vi "Untitled 1 (SubVI).vi"(5 "Sensor Data":string[][](array[string]), 6 "LDO Control Input":T3, 7 "Data Cluster":T5, 8 "error in (no error)":errorcluster, 9 "Ultramat 23":string[][](array[string]), 10 "Gross Heating Value, Vol (Real, Dry)":dbl, 11 "Header Array":string[](array[string])) -> (0 "error out":errorcluster, 2 "Gas Rate (BTU/hr)":dbl, 3 "Array":string[][](array[string]))   [LabVIEW 2020]
uses:
  Modbus LDO Control.ctl
  Drivers/Alicat LabVIEW Drivers 2v1/Sub-VIs/Data Cluster.ctl
  Modbus PLC Data All.ctl
  Modbus FVIR Control.ctl
  WritingDataFile/Data to Save.ctl
panel:
  in  "PLC Data Out":T1
  # "Totalizer Timer"
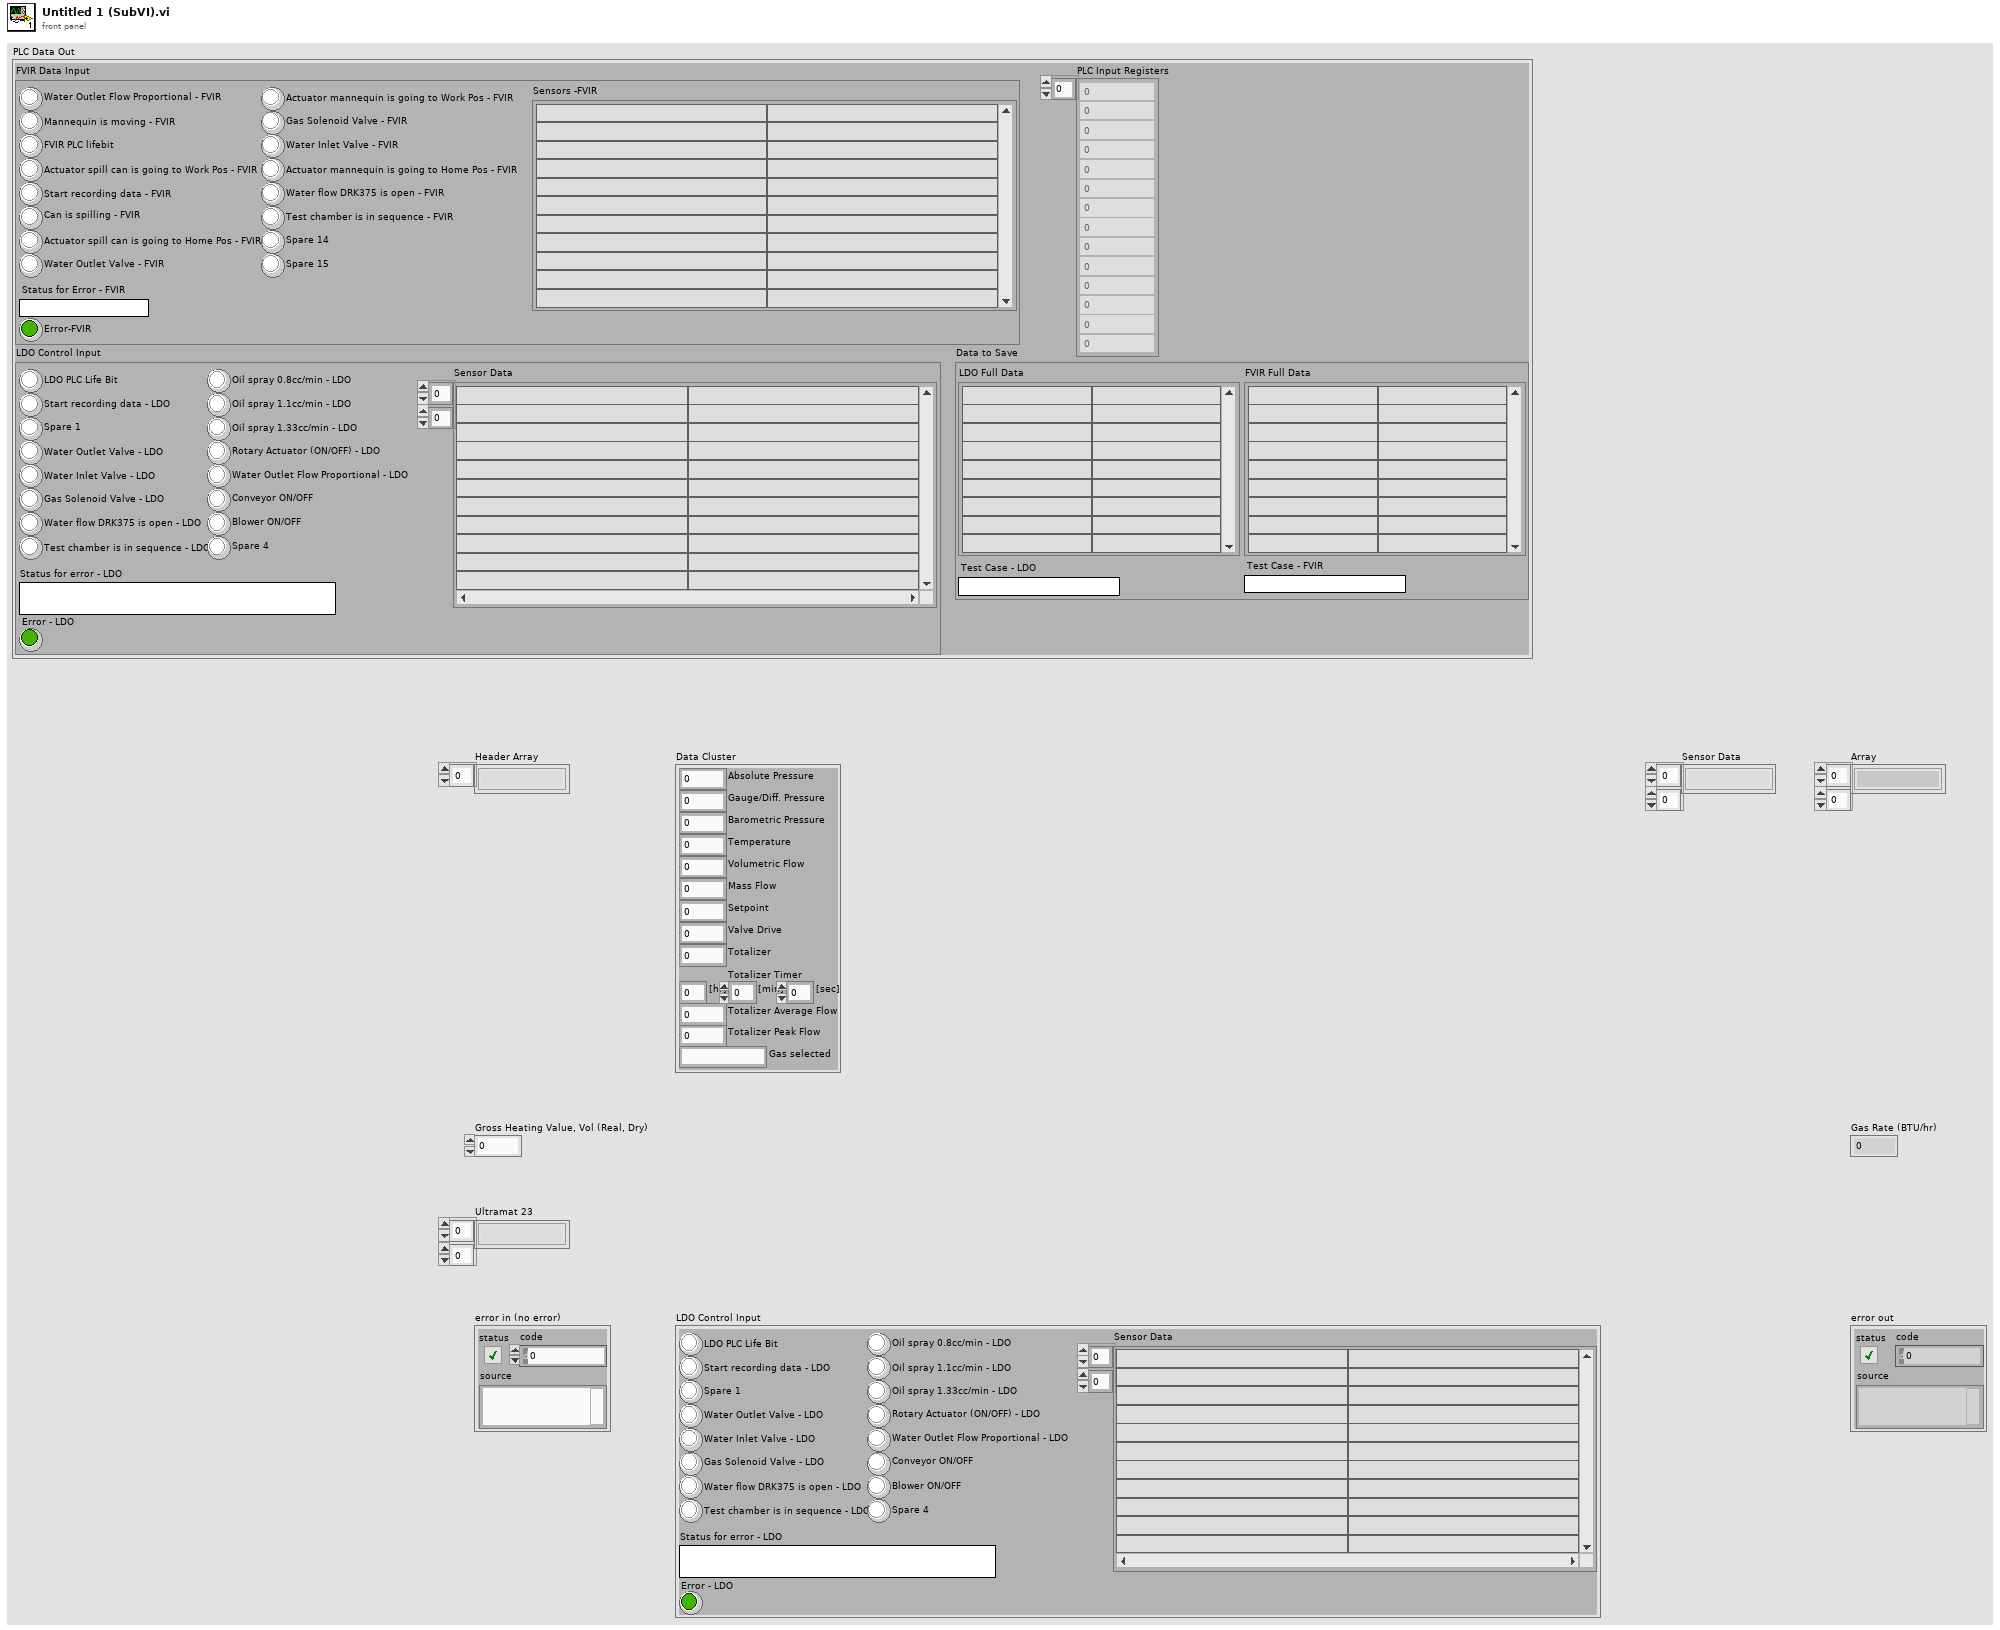
[diagram p1: front panel]
types:
  T1 = typedef "Modbus PLC Data All.ctl" = cluster{"FVIR Data Input":T2, "LDO Control Input":T3, "PLC Input Registers":u16[], "Data to Save":T4}
  T2 = typedef "Modbus FVIR Control.ctl" = cluster{"Spare 15":bool, "Spare 14":bool, "Actuator mannequin is going to Work Pos - FVIR":bool, "Actuator mannequin is going to Home Pos - FVIR":bool, "Test chamber is in sequence - FVIR ":bool, "Water flow DRK375 is open - FVIR":bool, "Gas Solenoid Valve - FVIR":bool, "Water Inlet Valve - FVIR":bool, "Water Outlet Flow Proportional - FVIR":bool, "Start recording data - FVIR":bool, "Actuator spill can is going to Work Pos - FVIR":bool, "Actuator spill can is going to Home Pos - FVIR":bool, "Water Outlet Valve - FVIR":bool, "Can is spilling - FVIR":bool, "Mannequin is moving - FVIR":bool, "FVIR PLC lifebit":bool, "Status for Error - FVIR":string, "Error-FVIR":bool, "Sensors -FVIR":string[][]}
  T3 = typedef "Modbus LDO Control.ctl" = cluster{"LDO PLC Life Bit":bool, "Start recording data - LDO":bool, "Spare 1":bool, "Water Outlet Valve - LDO":bool, "Water Inlet Valve - LDO":bool, "Gas Solenoid Valve - LDO":bool, "Water flow DRK375 is open - LDO":bool, "Test chamber is in sequence - LDO":bool, "Oil spray 0.8cc/min - LDO":bool, "Oil spray 1.1cc/min - LDO":bool, "Oil spray 1.33cc/min - LDO":bool, "Rotary Actuator (ON/OFF) - LDO":bool, "Water Outlet Flow Proportional - LDO":bool, "Conveyor ON/OFF":bool, "Blower ON/OFF":bool, "Spare 4":bool, "Status for error - LDO":string, "Error - LDO":bool, "Sensor Data":string[][]}
  T4 = typedef "Data to Save.ctl" = cluster{"LDO Full Data":string[][], "FVIR Full Data":string[][], "Test Case - FVIR":string, "Test Case - LDO":string}
  T5 = typedef "Data Cluster.ctl" = cluster{"Absolute Pressure":dbl, "Gauge/Diff. Pressure":dbl, "Barometric Pressure":dbl, "Temperature":dbl, "Volumetric Flow":dbl, "Mass Flow":dbl, "Setpoint":dbl, "Valve Drive":dbl, "Totalizer":dbl, "[hr]":dbl, "[min]":dbl, "[sec]":dbl, "Totalizer Average Flow":dbl, "Totalizer Peak Flow":dbl, "Gas selected":string}
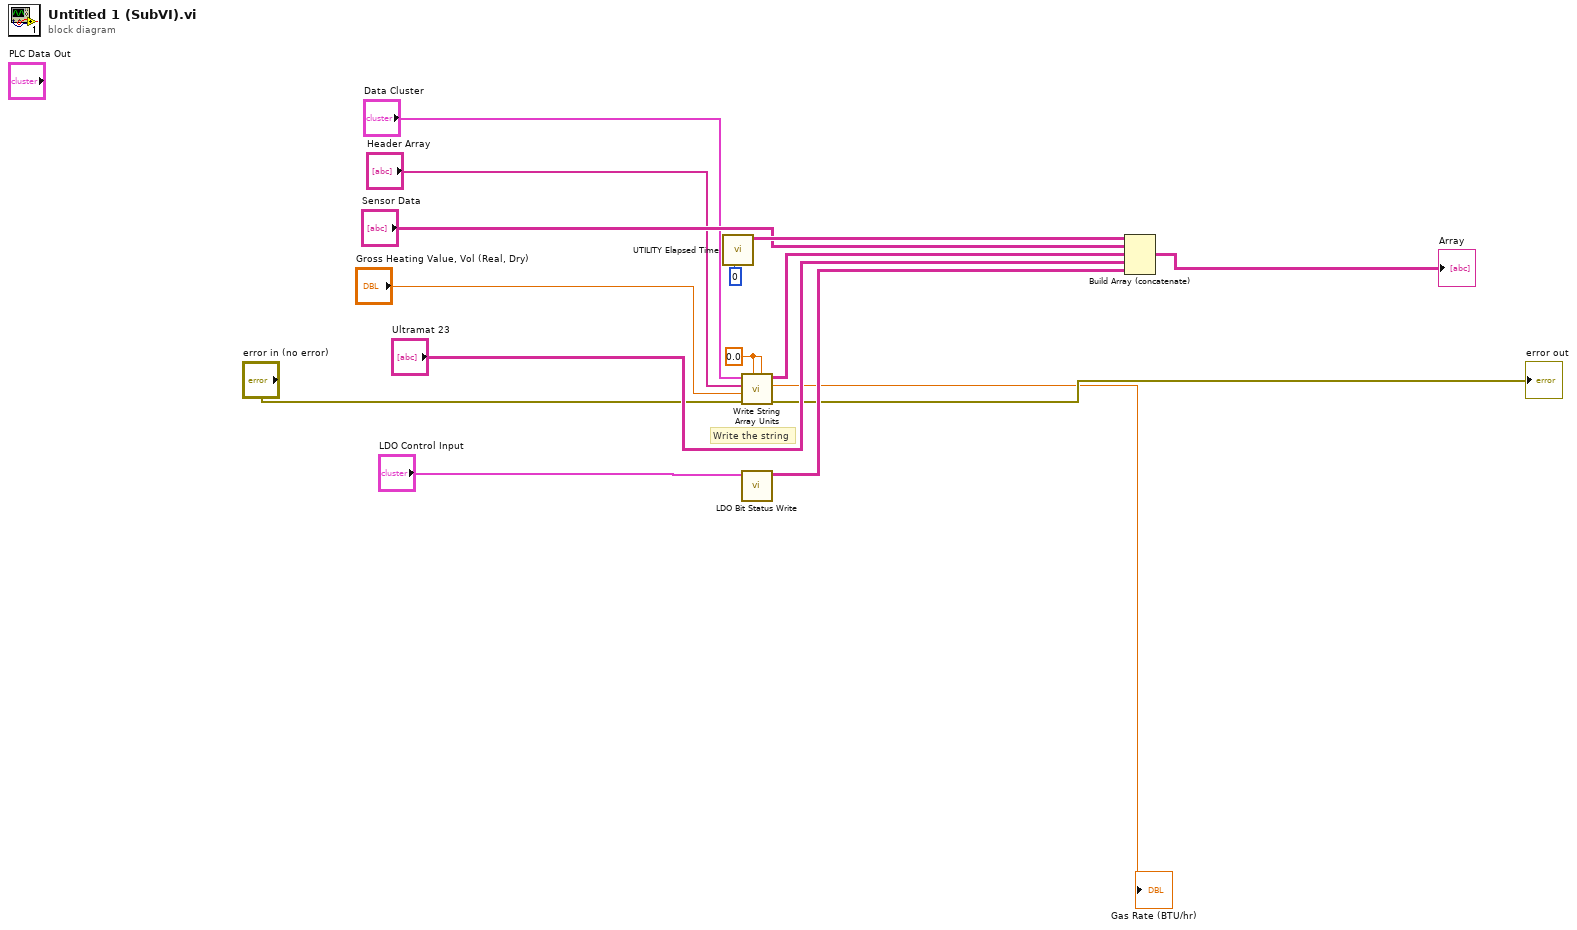
[diagram p0: block diagram]
diagram:
  w1 = 0.0 ("HHV_1")
  # "Write the string"
  n1 = call "UTILITY Elapsed Time.vi"("precision (6)"=i16 0) -> ("Total Array"=w14:string[][])  [unwired: 6 in, 4 out]
  n2 = call "Write String Array Units.vi"("Total_1"=w1, "HHV_1"=w1, "Error In"="error in (no error)", "Gross Heating Value, Vol (Real, Dry)"="Gross Heating Value, Vol (Real, Dry)", "Header Array"="Header Array", "Data Cluster"="Data Cluster") -> ("Error Out"=→"error out":errorcluster, "Gas Rate (BTU/hr)"=→"Gas Rate (BTU/hr)":dbl, "String Data"=w5:string[][])  [unwired: 3 in]
  n3 = call "LDO Bit Status Write.vi"("LDO Control Input"="LDO Control Input") -> ("Bit Status"=w13:string[][])  [unwired: 9 in, 1 out]
  n4 = Build Array (concatenate)(w14, "Sensor Data", w5, "Ultramat 23", w13) -> (→"Array":string[][])
